vi "Core.vi"(8 "error in (no error)":errorcluster, 10 "Actor in":refnum<class "Actor.lvclass">, 11 "Instrument Handler Response Msg in":refnum<class "Instrument Handler Response Msg.lvclass">) -> (0 "error out":errorcluster, 1 "Data":refnum<class "Data.lvclass">, 2 "Actor out":refnum<class "Actor.lvclass">, 3 "Instrument Handler Response Msg out":refnum<class "Instrument Handler Response Msg.lvclass">)   [LabVIEW 2020, in "Instrument Handler.lvlib" / "Instrument Handler Response Msg.lvclass"]
doc: "Core of the Reponse Msg. Put the active code here.\n\nThis implementation does nothing."
uses:
  Instrument Handler Response Msg.lvclass
  PPL/HDH.Data.Generic.lvlibp/Data.lvclass
  PPL/HDH.Actor Framework.Core.Actor.lvlibp/1abvi3w/vi.lib/ActorFramework/Actor/Actor.lvclass
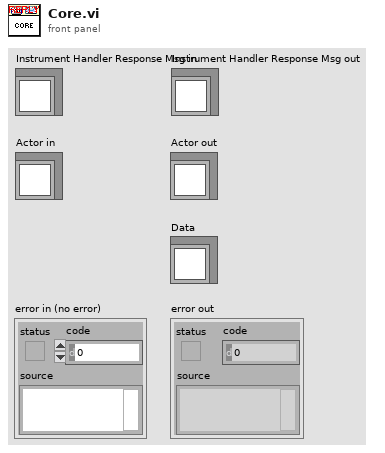
[diagram p1: front panel]
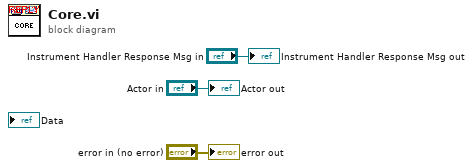
[diagram p0: block diagram]
diagram:
  "error out" <- "error in (no error)"
  "Actor out" <- "Actor in"
  "Instrument Handler Response Msg out" <- "Instrument Handler Response Msg in"
